vi "Update Build Version.vi"(8 "Error In":errorcluster, 11 "Target Project Root In":path) -> (0 "Error Out":errorcluster, 3 "Target Project Root Out":path)   [LabVIEW 2017, in "Scripts.lvlib"]
doc: "Copies the build specification from the target previous version, where the build version has been autoincremented, to the VIPB for the trunk/source project."
uses:
  Scripts.lvlib
  <vilib>/JKI/VIPM API/VIPM API_vipm_api.lvlib
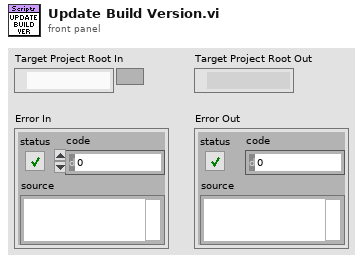
[diagram p1: front panel]
types:
  T1 = typedef "VIPM API_vipm_api.lvlib/VI Package Build Spec Data Cluster_vipm_api.ctl" = cluster{"Package Version":T2, "Product Name":string, "Company Name":string, "Author Name (Person or Company)":string, "Product Homepage (URL)":string, "Legal Copyright":string, "License Agreement Name":string, "Product Description Summary":string, "Product Description":string, "Release Notes - Change Log":string}
  T2 = typedef "VIPM API_vipm_api.lvlib/Version Info Cluster_vipm_api.ctl" = cluster{"major":u32, "minor":u32, "patch":u32, "build":u32}
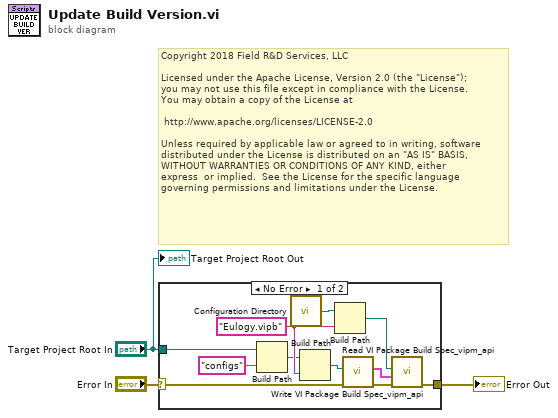
[diagram p0: block diagram]
diagram:
  # "Copyright 2018 Field R&D Services, LLC\n\nLicensed under the Apache License, Version 2.0 (the \"License\");\nyou may not use this file except in compliance with the License.\nYou may obtain a copy of the License at\n\n\thttp://www.apache.org/licenses/LICENSE-2.0\n\nUnless required by applicable law or agreed to in writing, software\ndistributed under the License is distributed on an \"AS IS\" BASIS,\nWITHOUT WARRANTIES OR CONDITIONS OF ANY KIND, either \nexpress  or implied.  See the License for the specific language \ngoverning permissions and limitations under the License."
  n1 = case shown="No Error" "Error In" {
    selector: "Error In" -> [w4 w15]
    tunnel: [w11 w15] -> w3
    tunnel: "Target Project Root In" -> [w5 _]
    frame No Error {
      w13 = "Eulogy.vipb" ("name or relative path")
      n2 = Build Path(base path=w5, name or relative path="configs") -> (appended path=w7:path)
      n3 = call "Configuration Directory.vi"() -> ("Configuration Directory"=w12:path)
      n4 = Build Path(base path=w7, name or relative path=w13) -> (appended path=w8:path)
      n5 = Build Path(base path=w12, name or relative path=w13) -> (appended path=w14:path)
      n6 = call <vilib>:"Read VI Package Build Spec_vipm_api.vi"("error in (no error)"=w4, "Path to VIPB File"=w8) -> ("error out"=w10:errorcluster, "VI Package Build Spec Data"=w9:T1)  [unwired: 8 in]
      n7 = call <vilib>:"Write VI Package Build Spec_vipm_api.vi"("error in (no error)"=w10, "VI Package Build Spec Data"=w9, "Path to VIPB File"=w14) -> ("error out"=w11:errorcluster)  [unwired: 8 in]
    }
    frame Error {
    }
  }
  "Error Out" <- w3
  "Target Project Root Out" <- "Target Project Root In"
